vi "PathPlanner_Trajectory_New.vi"(10 "StartingSpeeds":T5 {"vOmega" format="%10.3f"; "vY" format="%10.3f"; "vX" format="%10.3f"}, 11 "Path":T6={"Reversed"=FALSE, "RotationTargets"=[], "ConstraintZones"=[], "EventMarkers"=[], "GlobalConstraints"={"MaxVelocityMps;"=0.0, "MaxAccelerationMpsSq;"=0.0, "MaxAngularVelRadPsEc;"=0.0, "MaxAngularAccRadPSecSq"=0.0, "Exists"=FALSE, "Unlimited"=FALSE, "NominalVoltageVolts"=12.0}, "GoalEndState"={"VelocityMPS"=0.0, "Rotation"={"VALUE"=0.0, "COS"=1.0, "SIN"=0.0}}, "AllPoints"=[], "Name"="", "Waypoints"=[], "PointTowardsZones"=[], "IdealStartingState"={"VelocityMPS"=0.0, "Rotation"={"VALUE"=1.0, "COS"=0.0, "SIN"=0.0}, "NotNull"=FALSE}, "IsChoreoPath"=FALSE, "PreventFlipping"=FALSE} {"IdealStartingState"."Rotation"."SIN" format="%13.4f"; "IdealStartingState"."Rotation"."COS" format="%13.4f"; "IdealStartingState"."Rotation"."VALUE" format="%13.4f"; "PointTowardsZones"."TargetPosition"."Y" format="%14.3f"; "PointTowardsZones"."TargetPosition"."X" format="%14.3f"; "PointTowardsZones"."RotationOffset"."SIN" format="%13.4f"; "PointTowardsZones"."RotationOffset"."COS" format="%13.4f"; "PointTowardsZones"."RotationOffset"."VALUE" format="%13.4f"; "Waypoints"."nextControl"."Y" format="%14.3f"; "Waypoints"."nextControl"."X" format="%14.3f"; "Waypoints"."anchor"."Y" format="%14.3f"; "Waypoints"."anchor"."X" format="%14.3f"; "Waypoints"."prevControl"."Y" format="%14.3f"; "Waypoints"."prevControl"."X" format="%14.3f"; "AllPoints"."RotationTarget"."rotation"."SIN" format="%13.4f"; "AllPoints"."RotationTarget"."rotation"."COS" format="%13.4f"; "AllPoints"."RotationTarget"."rotation"."VALUE" format="%13.4f"; "AllPoints"."Position"."Y" format="%14.3f"; "AllPoints"."Position"."X" format="%14.3f"; "GoalEndState"."Rotation"."SIN" format="%13.4f"; "GoalEndState"."Rotation"."COS" format="%13.4f"; "GoalEndState"."Rotation"."VALUE" format="%13.4f"; "RotationTargets"."rotation"."SIN" format="%13.4f"; "RotationTargets"."rotation"."COS" format="%13.4f"; "RotationTargets"."rotation"."VALUE" format="%13.4f"}) -> (1 "PathPlannerTrajectoryEvents":T1, 3 "PathPlannerTrajectory":T18 {"States"."TargetHolonomicRotation"."SIN" format="%13.4f"; "States"."TargetHolonomicRotation"."COS" format="%13.4f"; "States"."TargetHolonomicRotation"."VALUE" format="%13.4f"; "States"."Heading"."SIN" format="%13.4f"; "States"."Heading"."COS" format="%13.4f"; "States"."Heading"."VALUE" format="%13.4f"; "States"."PositionMeters"."Y" format="%14.3f"; "States"."PositionMeters"."X" format="%14.3f"})   [LabVIEW 2019, in "PathPlanner24.lvlib"]
doc: "Generate a PathPlannerTrajectory\n\nInputs: \n - path - cluster - path to generate the trajectory for\n - startingSpeeds - chassis speeds - Starting speeds of the robot when starting the trajectory\n\nOutputs:\n - trajectory - cluster - created trajectory data\n - TrajectoryEvents - cluster - created trajectory events data cluster"
uses:
  PathPlanner24.lvlib
  TypeDef/PathPlannerCommandUtil.ctl
  TypeDef/PathPlannerTrajectoryEvent.ctl
  TypeDef/PathPlannerTrajectoryEvents.ctl
  ENum/PathPlanner_CommandUtil_Type_ENUM.ctl
  <vilib>/Rock Robotics/WPI/ThirdParty/JAS_Junk/TrajLib/TypeDef/ROTATION2D.ctl
  <vilib>/Rock Robotics/WPI/ThirdParty/JAS_Junk/TrajLib/Trajectory_Library.lvlib
  <vilib>/Rock Robotics/WPI/ThirdParty/JAS_Junk/TrajLib/TypeDef/TRANSLATION2D.ctl
  TypeDef/PathPlannerTrajectoryState.ctl
  TypeDef/PathPlannerTrajectory.ctl
  TypeDef/PathPlannerPathConstraints.ctl
  TypeDef/PathPlannerRotationTarget.ctl
  TypeDef/PathPlannerConstraintsZone.ctl
  TypeDef/PathPlannerEventMarker.ctl
  TypeDef/PathPlannerGoalEndState.ctl
  TypeDef/PathPlannerPathPoint.ctl
  TypeDef/PathPlannerPath.ctl
  <vilib>/Rock Robotics/WPI/ThirdParty/JAS_Junk/TrajLib/TypeDef/CHASSIS_SPEEDS.ctl
  TypeDef/PathPlannerWaypoint.ctl
  TypeDef/PathPlannerPointTowardsZone.ctl
  TypeDef/PathPlannerIdealStartingState.ctl
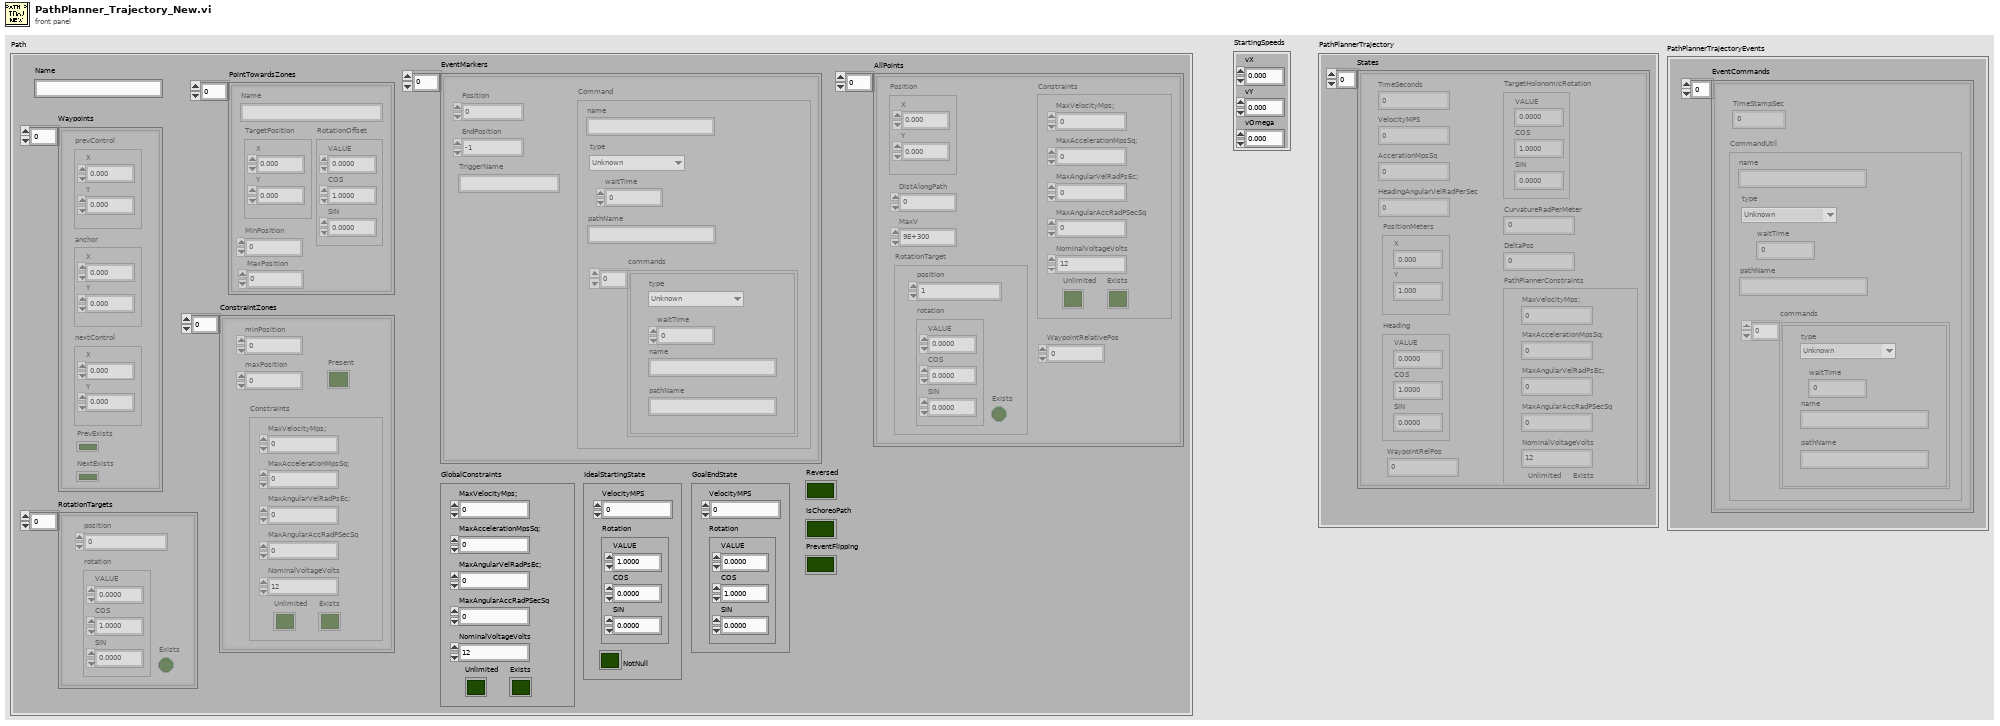
[diagram p1: front panel]
types:
  T1 = typedef "PathPlanner24.lvlib/PathPlannerTrajectoryEvents.ctl" = cluster{"EventCommands":T2[]}
  T2 = typedef "PathPlanner24.lvlib/PathPlannerTrajectoryEvent.ctl" = cluster{"TimeStampSec":dbl, "CommandUtil":T3}
  T3 = typedef "PathPlanner24.lvlib/PathPlannerCommandUtil.ctl" = cluster{"waitTime":dbl, "name":string, "pathName":string, "commands":cluster{"type":T4, "waitTime":dbl, "name":string, "pathName":string}[], "type":T4}
  T4 = typedef "PathPlanner24.lvlib/PathPlanner_CommandUtil_Type_ENUM.ctl" = enum16{"Unknown", "Wait", "Named", "Path", "Sequential", "Parallel", "Race", "Deadline", "PointTowardsZoneEnter", "PointTowardsZoneExit", "TriggerEventStart", "TriggerEventStop", "TriggerEventOneshot"}
  T5 = typedef "Trajectory_Library.lvlib/CHASSIS_SPEEDS.ctl" = cluster{"vX":dbl, "vY":dbl, "vOmega":dbl}
  T6 = typedef "PathPlanner24.lvlib/PathPlannerPath.ctl" = cluster{"Reversed":bool, "RotationTargets":T7[], "ConstraintZones":T9[], "EventMarkers":T11[], "GlobalConstraints":T10, "GoalEndState":T12, "AllPoints":T13[], "Name":string, "Waypoints":T15[], "PointTowardsZones":T16[], "IdealStartingState":T17, "IsChoreoPath":bool, "PreventFlipping":bool}
  T7 = typedef "PathPlanner24.lvlib/PathPlannerRotationTarget.ctl" = cluster{"position":dbl, "rotation":T8, "Exists":bool}
  T8 = typedef "Trajectory_Library.lvlib/ROTATION2D.ctl" = cluster{"VALUE":dbl, "COS":dbl, "SIN":dbl}
  T9 = typedef "PathPlanner24.lvlib/PathPlannerConstraintsZone.ctl" = cluster{"minPosition":dbl, "maxPosition":dbl, "Constraints":T10, "Present":bool}
  T10 = typedef "PathPlanner24.lvlib/PathPlannerPathConstraints.ctl" = cluster{"MaxVelocityMps;":dbl, "MaxAccelerationMpsSq;":dbl, "MaxAngularVelRadPsEc;":dbl, "MaxAngularAccRadPSecSq":dbl, "Exists":bool, "Unlimited":bool, "NominalVoltageVolts":dbl}
  T11 = typedef "PathPlanner24.lvlib/PathPlannerEventMarker.ctl" = cluster{"Position":dbl, "Command":T3, "TriggerName":string, "EndPosition":dbl}
  T12 = typedef "PathPlanner24.lvlib/PathPlannerGoalEndState.ctl" = cluster{"VelocityMPS":dbl, "Rotation":T8}
  T13 = typedef "PathPlanner24.lvlib/PathPlannerPathPoint.ctl" = cluster{"Position":T14, "DistAlongPath":dbl, "MaxV":dbl, "Constraints":T10, "RotationTarget":T7, "WaypointRelativePos":dbl}
  T14 = typedef "Trajectory_Library.lvlib/TRANSLATION2D.ctl" = cluster{"X":dbl, "Y":dbl}
  T15 = typedef "PathPlanner24.lvlib/PathPlannerWaypoint.ctl" = cluster{"prevControl":T14, "anchor":T14, "nextControl":T14, "PrevExists":bool, "NextExists":bool}
  T16 = typedef "PathPlanner24.lvlib/PathPlannerPointTowardsZone.ctl" = cluster{"RotationOffset":T8, "Name":string, "TargetPosition":T14, "MinPosition":dbl, "MaxPosition":dbl}
  T17 = typedef "PathPlanner24.lvlib/PathPlannerIdealStartingState.ctl" = cluster{"VelocityMPS":dbl, "Rotation":T8, "NotNull":bool}
  T18 = typedef "PathPlanner24.lvlib/PathPlannerTrajectory.ctl" = cluster{"States":T19[]}
  T19 = typedef "PathPlanner24.lvlib/PathPlannerTrajectoryState.ctl" = cluster{"TimeSeconds":dbl, "VelocityMPS":dbl, "AccerationMpsSq":dbl, "HeadingAngularVelRadPerSec":dbl, "PositionMeters":T14, "Heading":T8, "TargetHolonomicRotation":T8, "CurvatureRadPerMeter":dbl, "PathPlannerConstraints":T10, "DeltaPos":dbl, "WaypointRelPos":dbl}
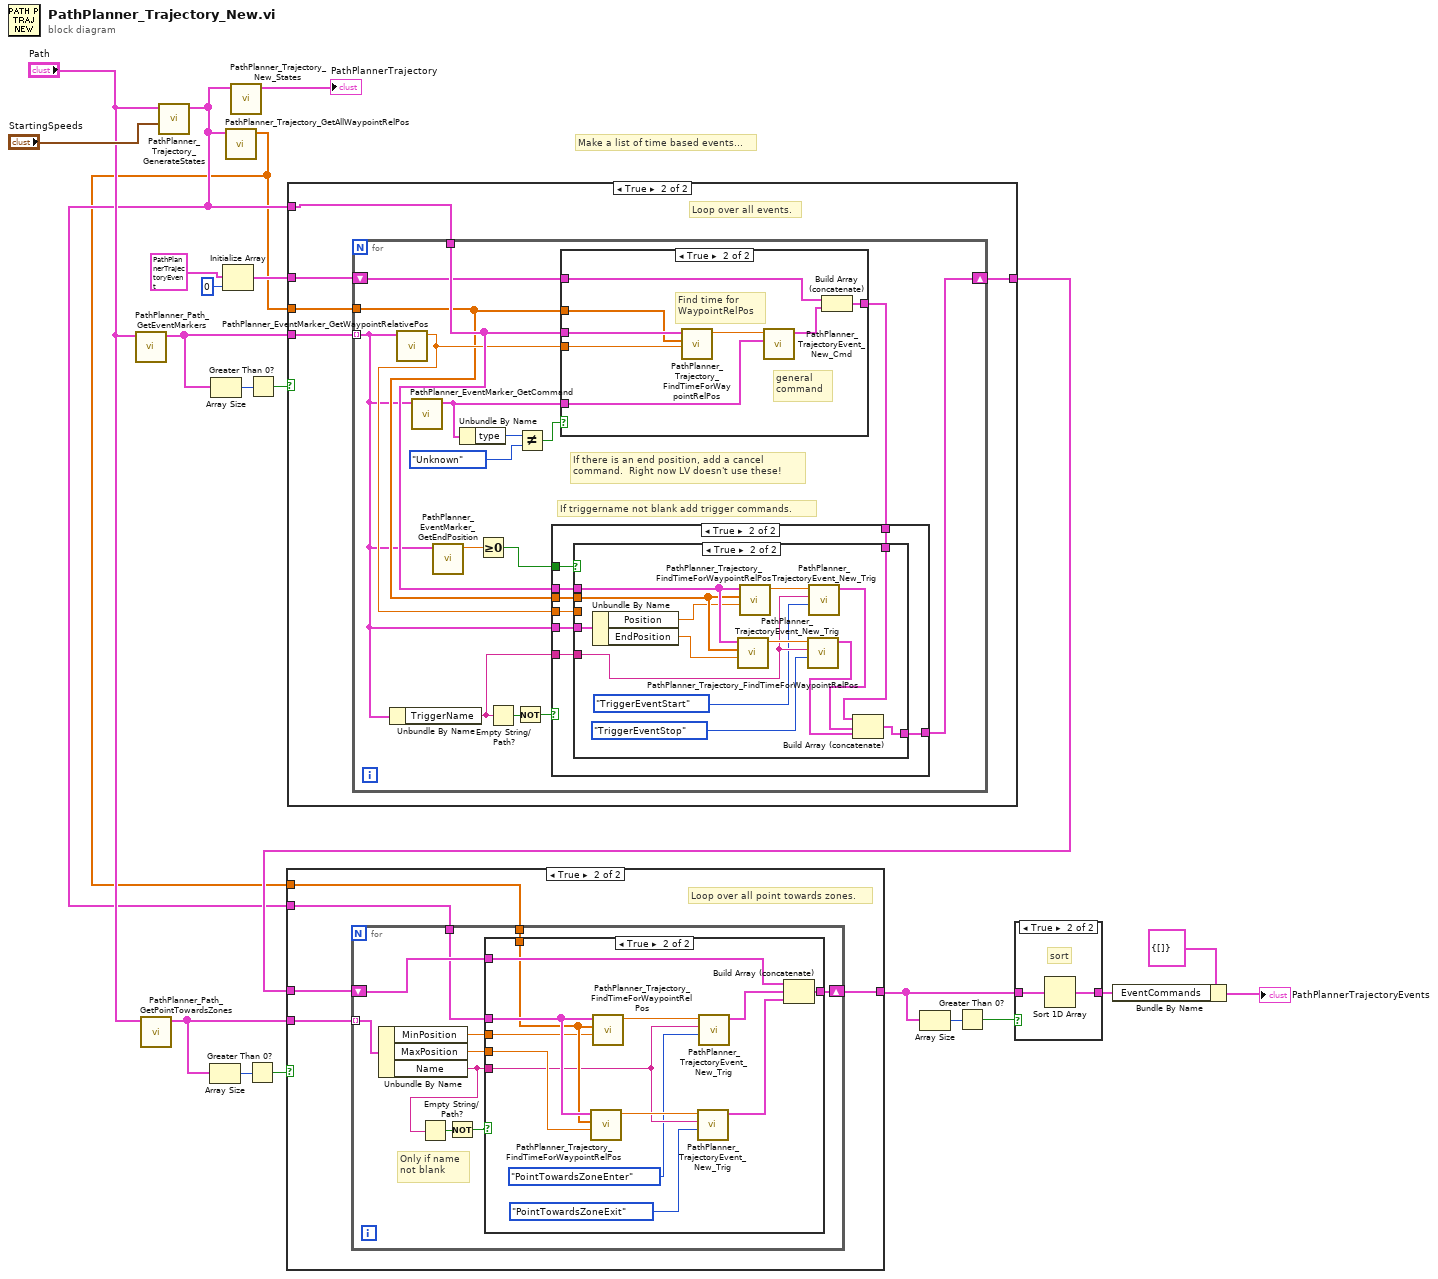
[diagram p0: block diagram]
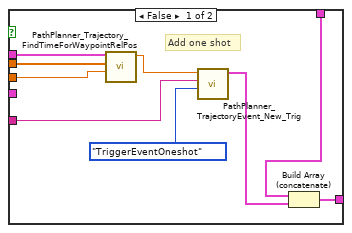
[diagram p7: hidden frame]
diagram:
  # "Make a list of time based events..."
  n1 = call "PathPlanner_Path_GetEventMarkers.vi"("PathPlannerPath"="Path") -> ("EventMarkers"=w18:T11[])  [unwired: 10 in]
  n2 = call "PathPlanner_Path_GetPointTowardsZones.vi"("PathPlannerPath"="Path") -> ("PointTowardsZones"=w8:T16[])  [unwired: 10 in]
  n3 = call "PathPlanner_Trajectory_GenerateStates.vi"("StartingSpeeds"="StartingSpeeds", "PathPlannerPath"="Path") -> ("PathPlannerStates"=w3:T19[])  [unwired: 9 in]
  n4 = Array Size(array=w8) -> (size(s)=w12:i32)
  n5 = Array Size(array=w18) -> (size(s)=w20:i32)
  n6 = Initialize Array(T2 {"TimeStampSec"=0.0, "CommandUtil"={"waitTime"=0.0, "name"="", "pathName"="", "commands"=[], "type"=enum."Unknown"}} ("TrajectoryEvent"), 0 ("dimension size")) -> (w15:T2[])
  n7 = call "PathPlanner_Trajectory_GetAllWaypointRelPos.vi"("PathPlannerStates"=w3) -> ("AllWaypointRelPos"=w1:dbl[])  [unwired: 10 in]
  n8 = call "PathPlanner_Trajectory_New_States.vi"("PathPlannerStates"=w3) -> ("PathPlannerTrajectory"=→"PathPlannerTrajectory":T18)  [unwired: 10 in]
  n9 = Greater Than 0?(x=w12) -> (x > 0?=w7:bool)
  n10 = Greater Than 0?(x=w20) -> (x > 0?=w19:bool)
  n11 = case shown="True" w19 {
    tunnel: [w22 w24] -> w10
    tunnel: w18 -> [_ w27]
    tunnel: w3 -> [_ w25]
    tunnel: w15 -> [w22 w26]
    tunnel: w1 -> [_ w23]
    frame False {
    }
    frame True {
      # "Loop over all events."
      n12 = for {
        shift-right: [w34] -> w24
        shift-left: w26 -> [w29]
        tunnel: w27 -> [w28] mode=indexing
        tunnel: w25 -> [w33]
        tunnel: w23 -> [w30]
        # "If triggername not blank add trigger commands."
        # "If there is an end position, add a cancel \ncommand.  Right now LV doesn't use these!"
        n13 = Unbundle By Name(w28) -> ("TriggerName"=w31:string)
        n14 = call "PathPlanner_EventMarker_GetWaypointRelativePos.vi"("in EventMarker"=w28) -> ("WaypointRelativePos"=w32:dbl)  [unwired: 10 in]
        n15 = call "PathPlanner_EventMarker_GetCommand.vi"("in EventMarker"=w28) -> ("Command"=w43:T3)  [unwired: 10 in]
        n16 = call "PathPlanner_EventMarker_GetEndPosition.vi"("in EventMarker"=w28) -> ("EndPosition"=w37:dbl)  [unwired: 10 in]
        n17 = Unbundle By Name(w43) -> ("type"=w42:T4)
        n18 = Greater Or Equal To 0?(x=w37) -> (x >= 0?=w36:bool)
        n19 = Empty String/Path?(string/path=w31) -> (empty?=w39:bool)
        n20 = Not(x=w39) -> (.not. x?=w38:bool)
        n21 = Not Equal?(x=w42, y=PathPlanner_CommandUtil_Type_ENUM."Unknown") -> (x != y?=w40:bool)
        n22 = case shown="True" w40 {
          tunnel: [w76 w83] -> w35
          tunnel: w33 -> [_ w82]
          tunnel: w32 -> [_ w81]
          tunnel: w43 -> [_ w79]
          tunnel: w30 -> [_ w78]
          tunnel: w29 -> [w76 w77]
          frame False {
          }
          frame True {
            # "Find time for \nWaypointRelPos"
            # "general \ncommand"
            n23 = call "PathPlanner_Trajectory_FindTimeForWaypointRelPos.vi"("WaypointRelPos"=w81, "AllWayPointRelPos"=w78, "PathPlannerStates"=w82) -> ("Time_Secs"=w80:dbl)  [unwired: 8 in]
            n24 = call "PathPlanner_TrajectoryEvent_New_Cmd.vi"("Command"=w79, "Time_Secs"=w80) -> ("TrajectoryEvent"=w84:T2)  [unwired: 9 in]
            n25 = Build Array (concatenate)(w77, w84) -> (w83:T2[])
          }
        }
        n26 = case shown="True" w38 {
          tunnel: w36 -> [_ w52]
          tunnel: w35 -> [w44 w47]
          tunnel: [w44 w46] -> w34
          tunnel: w30 -> [_ w51]
          tunnel: w33 -> [_ w50]
          tunnel: w32 -> [_ w49]
          tunnel: w31 -> [_ w48]
          tunnel: w28 -> [_ w45]
          frame False {
          }
          frame True {
            n27 = case shown="True" w52 {
              tunnel: w51 -> [w61 w71]
              tunnel: w50 -> [w60 w72]
              tunnel: w49 -> [w59 _]
              tunnel: w48 -> [w57 w68]
              tunnel: w47 -> [w56 w66]
              tunnel: [w54 w67] -> w46
              tunnel: w45 -> [_ w73]
              frame False {
                # "Add one shot"
                n28 = call "PathPlanner_Trajectory_FindTimeForWaypointRelPos.vi"("WaypointRelPos"=w59, "AllWayPointRelPos"=w61, "PathPlannerStates"=w60) -> ("Time_Secs"=w58:dbl)  [unwired: 8 in]
                n29 = call "PathPlanner_TrajectoryEvent_New_Trig.vi"("Cmd Type"=PathPlanner_CommandUtil_Type_ENUM."TriggerEventOneshot" ("CommandUtil.type"), "Cmd Name"=w57, "Time_Secs"=w58) -> ("TrajectoryEvent"=w55:T2)  [unwired: 8 in]
                n30 = Build Array (concatenate)(w56, w55) -> (w54:T2[])
              }
              frame True {
                n31 = Unbundle By Name(w73) -> ("Position"=w70:dbl, "EndPosition"=w69:dbl)
                n32 = call "PathPlanner_Trajectory_FindTimeForWaypointRelPos.vi"("WaypointRelPos"=w69, "AllWayPointRelPos"=w71, "PathPlannerStates"=w72) -> ("Time_Secs"=w74:dbl)  [unwired: 8 in]
                n33 = call "PathPlanner_Trajectory_FindTimeForWaypointRelPos.vi"("WaypointRelPos"=w70, "AllWayPointRelPos"=w71, "PathPlannerStates"=w72) -> ("Time_Secs"=w75:dbl)  [unwired: 8 in]
                n34 = call "PathPlanner_TrajectoryEvent_New_Trig.vi"("Cmd Type"=PathPlanner_CommandUtil_Type_ENUM."TriggerEventStop" ("CommandUtil.type"), "Cmd Name"=w68, "Time_Secs"=w74) -> ("TrajectoryEvent"=w64:T2)  [unwired: 8 in]
                n35 = call "PathPlanner_TrajectoryEvent_New_Trig.vi"("Cmd Type"=PathPlanner_CommandUtil_Type_ENUM."TriggerEventStart" ("CommandUtil.type"), "Cmd Name"=w68, "Time_Secs"=w75) -> ("TrajectoryEvent"=w65:T2)  [unwired: 8 in]
                n36 = Build Array (concatenate)(w66, w65, w64) -> (w67:T2[])
              }
            }
          }
        }
      }
    }
  }
  n37 = case shown="True" w7 {
    tunnel: [w85 w87] -> w5
    tunnel: w8 -> [_ w90]
    tunnel: w3 -> [_ w88]
    tunnel: w10 -> [w85 w89]
    tunnel: w1 -> [_ w86]
    frame False {
    }
    frame True {
      # "Loop over all point towards zones."
      n38 = for {
        shift-right: [w99] -> w87
        shift-left: w89 -> [w100]
        tunnel: w90 -> [w98] mode=indexing
        tunnel: w88 -> [w97]
        tunnel: w86 -> [w96]
        # "Only if name\nnot blank"
        n39 = Unbundle By Name(w98) -> ("MinPosition"=w95:dbl, "MaxPosition"=w94:dbl, "Name"=w91:string)
        n40 = Empty String/Path?(string/path=w91) -> (empty?=w93:bool)
        n41 = Not(x=w93) -> (.not. x?=w92:bool)
        n42 = case shown="True" w92 {
          tunnel: w100 -> [w101 w114]
          tunnel: [w101 w113] -> w99
          tunnel: w97 -> [_ w112]
          tunnel: w96 -> [_ w111]
          tunnel: w95 -> [_ w110]
          tunnel: w94 -> [_ w109]
          tunnel: w91 -> [_ w106]
          frame False {
          }
          frame True {
            n43 = call "PathPlanner_Trajectory_FindTimeForWaypointRelPos.vi"("WaypointRelPos"=w109, "AllWayPointRelPos"=w111, "PathPlannerStates"=w112) -> ("Time_Secs"=w107:dbl)  [unwired: 8 in]
            n44 = call "PathPlanner_Trajectory_FindTimeForWaypointRelPos.vi"("WaypointRelPos"=w110, "AllWayPointRelPos"=w111, "PathPlannerStates"=w112) -> ("Time_Secs"=w108:dbl)  [unwired: 8 in]
            n45 = call "PathPlanner_TrajectoryEvent_New_Trig.vi"("Cmd Type"=PathPlanner_CommandUtil_Type_ENUM."PointTowardsZoneExit" ("CommandUtil.type"), "Cmd Name"=w106, "Time_Secs"=w107) -> ("TrajectoryEvent"=w102:T2)  [unwired: 8 in]
            n46 = call "PathPlanner_TrajectoryEvent_New_Trig.vi"("Cmd Type"=PathPlanner_CommandUtil_Type_ENUM."PointTowardsZoneEnter" ("CommandUtil.type"), "Cmd Name"=w106, "Time_Secs"=w108) -> ("TrajectoryEvent"=w103:T2)  [unwired: 8 in]
            n47 = Build Array (concatenate)(w114, w103, w102) -> (w113:T2[])
          }
        }
      }
    }
  }
  n48 = Array Size(array=w5) -> (size(s)=w6:i32)
  n49 = Greater Than 0?(x=w6) -> (x > 0?=w4:bool)
  n50 = case shown="True" w4 {
    tunnel: w5 -> [w115 w117]
    tunnel: [w115 w116] -> w9
    frame False {
    }
    frame True {
      # "sort"
      n51 = Sort 1D Array(array=w117) -> (sorted array=w116:T2[])
    }
  }
  n52 = Bundle By Name(cluster=T1 {"EventCommands"=[]} ("PathPlannerTrajectoryEvents"), "EventCommands"=w9) -> (→"PathPlannerTrajectoryEvents":T1)
